vi "p1.vi"() -> ()   [LabVIEW 2023, in "d17.lvlib"]
uses:
  d17.lvlib
  AOC/AOC.lvlib
panel:
  out "Intensity Graph":dbl[][](graph)
  out "min value":u16
  in  "Example":string="2413432311323\n3215453535623\n3255245654254\n3446585845452\n4546657867536\n1438598798454\n4457876987766\n3637877979653\n4654967986887\n4564679986453\n1224686865563\n2546548887735\n4322674655533"
  in  "Example":bool
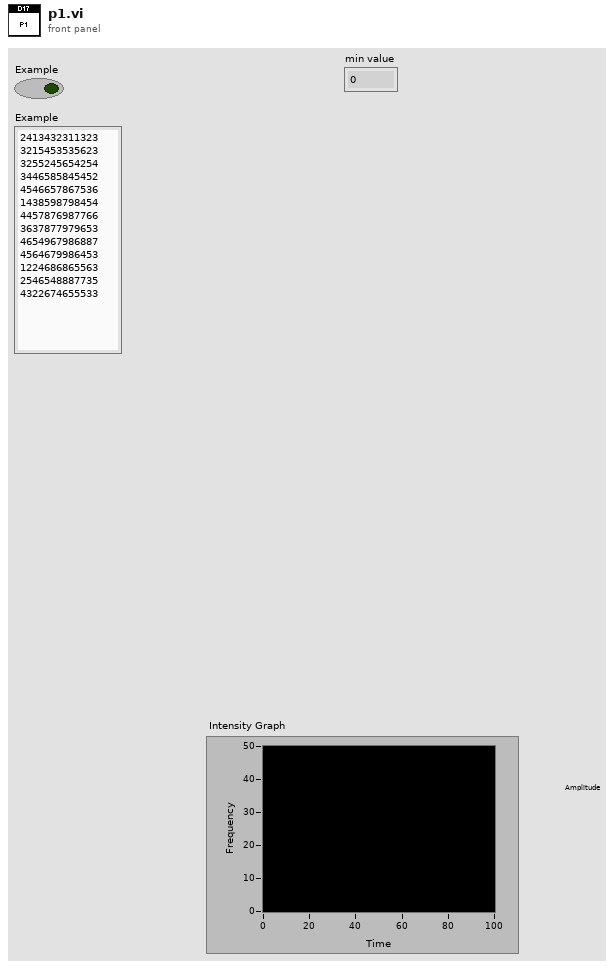
[diagram p1: front panel]
types:
  T1 = map{cluster{"unsigned 8bit integer":i16, "unsigned 8bit integer":i16}, cluster{"unsigned 8bit integer":i16, "unsigned 8bit integer":i16}[]}
  T2 = cluster{"heat loss":u16, "position":cluster{"unsigned 8bit integer":i16, "unsigned 8bit integer":i16}, "direction":cluster{"unsigned 8bit integer":i16, "unsigned 8bit integer":i16}}
  T3 = cluster{"unsigned 8bit integer":i16, "unsigned 8bit integer":i16}
  T4 = map{cluster{cluster{"unsigned 8bit integer":i16, "unsigned 8bit integer":i16}, "RIGHT":cluster{"unsigned 8bit integer":i16, "unsigned 8bit integer":i16}}, u16}
  T5 = cluster{cluster{"unsigned 8bit integer":i16, "unsigned 8bit integer":i16}, "RIGHT":cluster{"unsigned 8bit integer":i16, "unsigned 8bit integer":i16}}
  T6 = cluster{cluster{"unsigned 8bit integer":i16, "unsigned 8bit integer":i16}, "LEFT":cluster{"unsigned 8bit integer":i16, "unsigned 8bit integer":i16}}
  T7 = cluster{cluster{"unsigned 8bit integer":i16, "unsigned 8bit integer":i16}, "UP":cluster{"unsigned 8bit integer":i16, "unsigned 8bit integer":i16}}
  T8 = cluster{cluster{"unsigned 8bit integer":i16, "unsigned 8bit integer":i16}, "DOWN":cluster{"unsigned 8bit integer":i16, "unsigned 8bit integer":i16}}
  T9 = cluster{cluster{"unsigned 8bit integer":i16, "unsigned 8bit integer":i16}, "DOWN":cluster{"unsigned 8bit integer":i16, "unsigned 8bit integer":i16}}[]
  T10 = cluster{"unsigned 8bit integer":i16, "unsigned 8bit integer":i16}[]
  T11 = cluster{"position":cluster{"unsigned 8bit integer":i16, "unsigned 8bit integer":i16}, "direction":cluster{"unsigned 8bit integer":i16, "unsigned 8bit integer":i16}}
  T12 = cluster{u16, cluster{"unsigned 8bit integer":i16, "unsigned 8bit integer":i16}, "RIGHT":cluster{"unsigned 8bit integer":i16, "unsigned 8bit integer":i16}}
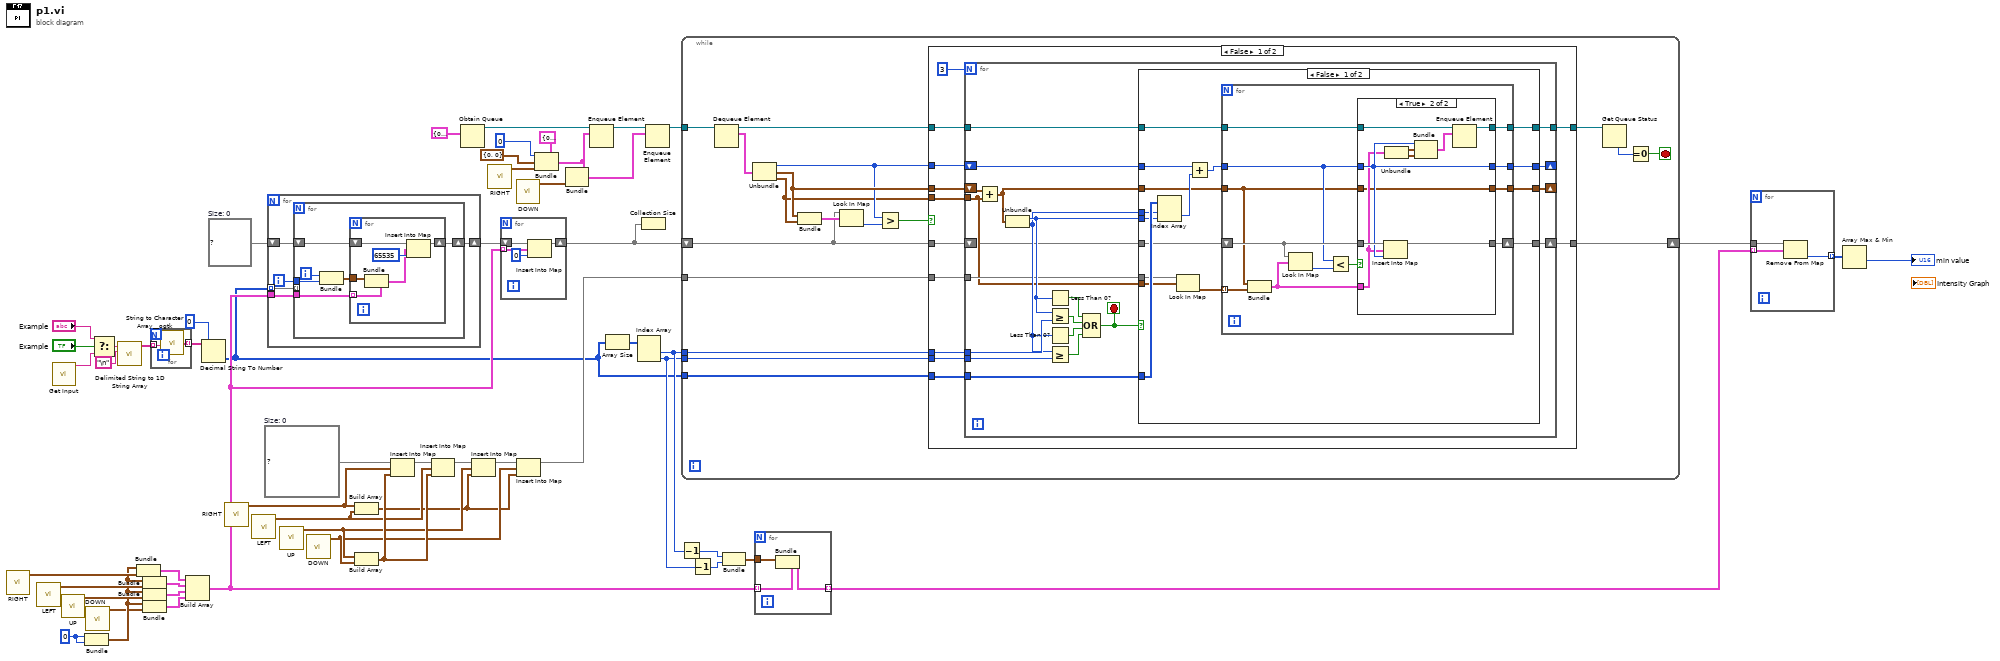
[diagram p0: block diagram]
diagram:
  w34 = T1 {}  # Size: 0
  w52 = i16 0 ("unsigned 8bit integer")
  w17 = T4 {}  # Size: 0
  n1 = call "RIGHT.vi"() -> ("RIGHT"=w51:T3)  [unwired: 11 in]
  n2 = call "LEFT.vi"() -> ("LEFT"=w50:T3)  [unwired: 11 in]
  n3 = call "Get Input.vi"() -> ("Input"=w55:string)  [unwired: 11 in]
  n4 = call "UP.vi"() -> ("UP"=w49:T3)  [unwired: 11 in]
  n5 = Bundle("unsigned 8bit integer"=w52, "unsigned 8bit integer"=w52) -> (w48:T3)  [unwired: 1 in]
  n6 = call "DOWN.vi"() -> ("DOWN"=w47:T3)  [unwired: 11 in]
  n7 = Select(t="Example", s="Example", f=w55) -> (s? t:f=w11:string)
  n8 = call <vilib>:"Delimited String to 1D String Array.vi"("delimiter"="\n", "delimited string"=w11) -> ("string array"=w8:string[])  [unwired: 9 in]
  n9 = Bundle(w48, "RIGHT"=w51) -> (w16:T5)  [unwired: 1 in]
  n10 = Bundle(w48, "LEFT"=w50) -> (w15:T6)  [unwired: 1 in]
  n11 = Bundle(w48, "UP"=w49) -> (w14:T7)  [unwired: 1 in]
  n12 = Bundle(w48, "DOWN"=w47) -> (w13:T8)  [unwired: 1 in]
  n13 = for {
    tunnel: w8 -> [w57] mode=indexing
    tunnel: [w56] -> w9 mode=indexing
    n14 = call <userlib>:"String to Character Array__ogtk.vi"("Input String"=w57) -> ("Character Array"=w56:string[])
  }
  n15 = Build Array(w16, w15, w14, w13) -> (w4:T9)
  n16 = Decimal String To Number(string=w9, default (0L)=i16 0 ("default (0 I32)")) -> (number=w2:i16[][])  [unwired: 1 in, 1 out]
  n17 = call "RIGHT.vi"() -> ("RIGHT"=w30:T3)  [unwired: 11 in]
  n18 = call "LEFT.vi"() -> ("LEFT"=w29:T3)  [unwired: 11 in]
  n19 = for {
    shift-right: [w60] -> w12
    shift-left: w17 -> [w62]
    tunnel: w2 -> [w58] mode=indexing
    tunnel: w4 -> [w59]
    i -> [w61]
    n20 = for {
      shift-right: [w66] -> w60
      shift-left: w62 -> [w65]
      tunnel: w61 -> [w67]
      tunnel: w59 -> [w64]
      tunnel: w58 -> [_] mode=indexing
      i -> [w68]
      n21 = Bundle(w68, w67) -> (w63:cluster{i32, i32})  [unwired: 1 in]
      n22 = for {
        tunnel: w64 -> [w73] mode=indexing
        shift-right: [w74] -> w66
        shift-left: w65 -> [w72]
        tunnel: w63 -> [w69]
        n23 = Bundle(cluster=w73, w69) -> (w70:T8)  [unwired: 1 in]
        n24 = Insert Into Map(map in=w72, key=w70, value=u16 65535) -> (map out=w74:T4)  [unwired: 2 out]
      }
    }
  }
  n25 = call "UP.vi"() -> ("UP"=w28:T3)  [unwired: 11 in]
  n26 = call "DOWN.vi"() -> ("DOWN"=w26:T3)  [unwired: 11 in]
  n27 = Build Array(w30, w29) -> (w25:T10)
  n28 = Build Array(w28, w26) -> (w32:T10)
  n29 = Insert Into Map(map in=w34, key=w30, value=w32) -> (map out=w33:T1)  [unwired: 2 out]
  n30 = Insert Into Map(map in=w33, key=w29, value=w32) -> (map out=w31:T1)  [unwired: 2 out]
  n31 = Obtain Queue(element data type=T2 {"heat loss"=0, "position"={"unsigned 8bit integer"=0, "unsigned 8bit integer"=0}, "direction"={"unsigned 8bit integer"=0, "unsigned 8bit integer"=0}} ("cluster")) -> (queue out=w41:refnum<queue>)  [unwired: 4 in, 2 out]
  n32 = Insert Into Map(map in=w31, key=w28, value=w25) -> (map out=w27:T1)  [unwired: 2 out]
  n33 = call "RIGHT.vi"() -> ("RIGHT"=w46:T3)  [unwired: 11 in]
  n34 = for {
    tunnel: w4 -> [w77] mode=indexing
    shift-right: [w78] -> w3
    shift-left: w12 -> [w76]
    n35 = Insert Into Map(map in=w76, key=w77, value=u16 0) -> (map out=w78:T4)  [unwired: 2 out]
  }
  n36 = call "DOWN.vi"() -> ("DOWN"=w39:T3)  [unwired: 11 in]
  n37 = Insert Into Map(map in=w27, key=w26, value=w25) -> (map out=w24:T1)  [unwired: 2 out]
  n38 = Bundle(cluster=T2 {"heat loss"=0, "position"={"unsigned 8bit integer"=0, "unsigned 8bit integer"=0}, "direction"={"unsigned 8bit integer"=0, "unsigned 8bit integer"=0}}, "heat loss"=u16 0 ("value"), "position"=T3 {"unsigned 8bit integer"=0, "unsigned 8bit integer"=0} ("output cluster"), "direction"=w46) -> (w40:T2)
  n39 = Bundle(cluster=w40, "direction"=w39) -> (w38:T2)  [unwired: 2 in]
  n40 = Enqueue Element(queue=w41, element=w40) -> (queue out=w37:refnum<queue>)  [unwired: 2 in, 2 out]
  n41 = Array Size(array=w2) -> (size(s)=w35:i32[])
  n42 = Index Array(array=w35) -> (element #1=w23:i32, element #2=w22:i32)  [unwired: 2 in]
  n43 = Collection Size(1:w3) -> ()  [unwired: 1 out]
  n44 = Enqueue Element(queue=w37, element=w38) -> (queue out=w36:refnum<queue>)  [unwired: 2 in, 2 out]
  n45 = Decrement(x=w23) -> (x-1=w21:i32)
  n46 = while {
    tunnel: w36 -> [w94]
    tunnel: w23 -> [w89]
    tunnel: w22 -> [w88]
    tunnel: w2 -> [w87]
    tunnel: w24 -> [w84]
    shift-right: [w82] -> w1
    shift-left: w3 -> [w83]
    stop <- w95 stop-if-true
    n47 = Dequeue Element(queue=w94) -> (queue out=w81:refnum<queue>, element=w93:T2)  [unwired: 2 in, 2 out]
    n48 = Unbundle(w93) -> ("heat loss"=w86:u16, "position"=w90:T3, "direction"=w85:T3)
    n49 = Bundle("position"=w90, "direction"=w85) -> (w92:T11)  [unwired: 1 in]
    n50 = Look In Map(map=w83, key=w92) -> (value=w91:u16)  [unwired: 1 in, 1 out]
    n51 = Greater?(x=w86, y=w91) -> (0:w79:bool)
    n52 = case shown="False" w79 {
      tunnel: w90 -> [w108 _]
      tunnel: w85 -> [w106 _]
      tunnel: w89 -> [w105 _]
      tunnel: w88 -> [w104 _]
      tunnel: w87 -> [w103 _]
      tunnel: w86 -> [w102 _]
      tunnel: w84 -> [w101 _]
      tunnel: w83 -> [w100 w177]
      tunnel: [w99 w177] -> w82
      tunnel: w81 -> [w98 w176]
      tunnel: [w97 w176] -> w80
      frame False {
        n53 = for {
          N: 3 -> [_]
          tunnel: w106 -> [w115]
          tunnel: w105 -> [w128]
          tunnel: w104 -> [w127]
          tunnel: w103 -> [w121]
          shift-right: [w117] -> _
          shift-left: w102 -> [w118]
          tunnel: w101 -> [w116]
          shift-right: [w112] -> w99
          shift-left: w100 -> [w114]
          tunnel: w98 -> [w111]
          tunnel: [w110] -> w97
          shift-right: [w109] -> _
          shift-left: w108 -> [w129]
          stop <- w122 stop-if-true
          n54 = Add(x=w129, y=w115) -> (x+y=w113:T3)
          n55 = Unbundle(w113) -> ("unsigned 8bit integer"=w120:i16, "unsigned 8bit integer"=w119:i16)
          n56 = Less Than 0?(x=w120) -> (x < 0?=w126:bool)
          n57 = Greater Or Equal?(x=w120, y=w128) -> (x >= y?=w125:bool)
          n58 = Less Than 0?(x=w119) -> (x < 0?=w124:bool)
          n59 = Greater Or Equal?(x=w119, y=w127) -> (x >= y?=w123:bool)
          n60 = Compound Arithmetic op=OR(w126, w125, w124, w123) -> (w122:bool)
          n61 = case shown="False" w122 {
            tunnel: w121 -> [w145 _]
            tunnel: w120 -> [w144 _]
            tunnel: w119 -> [w136 _]
            tunnel: w118 -> [w143 w175]
            tunnel: [w131 w175] -> w117
            tunnel: w115 -> [w141 _]
            tunnel: w116 -> [w140 _]
            tunnel: w114 -> [w137 w174]
            tunnel: w113 -> [w135 w172]
            tunnel: [w134 w174] -> w112
            tunnel: w111 -> [w133 w173]
            tunnel: [w132 w173] -> w110
            tunnel: [w130 w172] -> w109
            frame False {
              n62 = Index Array(array=w145, index (row)=w136, index (col)=w144) -> (element=w142:i16)
              n63 = Look In Map(map=w140, key=w141) -> (value=w139:T10)  [unwired: 1 in, 1 out]
              n64 = Add(x=w143, y=w142) -> (x+y=w138:u16)
              n65 = for {
                tunnel: w139 -> [w157] mode=indexing
                tunnel: w138 -> [w154]
                tunnel: w135 -> [w147]
                shift-right: [w152] -> w134
                shift-left: w137 -> [w155]
                tunnel: w133 -> [w151]
                tunnel: [w150] -> w132
                tunnel: [w149] -> w131
                tunnel: [w146] -> w130
                n66 = Bundle(w147, "RIGHT"=w157) -> (w153:T5)  [unwired: 1 in]
                n67 = Look In Map(map=w155, key=w153) -> (value=w156:u16)  [unwired: 1 in, 1 out]
                n68 = Less?(x=w154, y=w156) -> (x < y?=w148:bool)
                n69 = case shown="True" w148 {
                  tunnel: w155 -> [w161 w171]
                  tunnel: w154 -> [w159 w167]
                  tunnel: w153 -> [_ w166]
                  tunnel: [w161 w170] -> w152
                  tunnel: w151 -> [w160 w169]
                  tunnel: [w160 w168] -> w150
                  tunnel: [w159 w167] -> w149
                  tunnel: w147 -> [w158 w162]
                  tunnel: [w158 w162] -> w146
                  frame False {
                  }
                  frame True {
                    n70 = Insert Into Map(map in=w171, key=w166, value=w167) -> (map out=w170:T4)  [unwired: 2 out]
                    n71 = Unbundle(w166) -> (w165:T3, "RIGHT"=w164:T3)
                    n72 = Bundle(w167, w165, "RIGHT"=w164) -> (w163:T12)  [unwired: 1 in]
                    n73 = Enqueue Element(queue=w169, element=w163) -> (queue out=w168:refnum<queue>)  [unwired: 2 in, 2 out]
                  }
                }
              }
            }
            frame True {
            }
          }
        }
      }
      frame True {
      }
    }
    n74 = Get Queue Status(queue=w80) -> (# elements in queue=w96:i32)  [unwired: 2 in, 7 out]
    n75 = Equal To 0?(x=w96) -> (x = 0?=w95:bool)
  }
  n76 = Decrement(x=w22) -> (x-1=w20:i32)
  n77 = Bundle(w21, w20) -> (w5:cluster{i32, i32})  [unwired: 1 in]
  n78 = for {
    tunnel: [w179] -> w6 mode=indexing
    tunnel: w4 -> [w180] mode=indexing
    tunnel: w5 -> [w178]
    n79 = Bundle(cluster=w180, w178) -> (w179:T8)  [unwired: 1 in]
  }
  n80 = for {
    tunnel: w1 -> [w183]
    tunnel: w6 -> [w182] mode=indexing
    tunnel: [w181] -> w19 mode=indexing
    n81 = Remove From Map(10:w182, 11:w183) -> (1:w181:u16)  [unwired: 2 out]
  }
  n82 = Array Max & Min(array=w19) -> (min value=→"min value":u16)  [unwired: 3 out]
